vi "ni579x Wait for EEPROM Operation.vi"(0 "Register Bus":T1, 1 "scope":string(combo)="characterization data eeprom", 9 "timeout [s]":dbl=10.0, 11 "Error In":errorcluster) -> (4 "Register Bus (out)":T1, 15 "Error Out":errorcluster)   [LabVIEW 2015, in "ni579x Config v2 Host.lvlib"]
uses:
  <instrlib>/ni579x/Config/v2/Host/ni579x Config v2 Host.lvlib
  <instrlib>/_niInstr/Register Bus/v0/Host/Public/Register Bus Session.ctl
  <instrlib>/_niInstr/Register Bus/v0/Host/Private/Session Data.ctl
  <instrlib>/ni579x/Config/v2/Shared/Types/ni579x FAM Register Offset.ctl
  <instrlib>/ni579x/Config/v2/Shared/Types/ni579x FAM Register Operation.ctl
  <instrlib>/ni579x/Config/v2/Shared/ni579x Config v2 Shared.lvlib
  <instrlib>/_niInstr/Register Bus/v0/Host/niInstr Register Bus v0 Host.lvlib
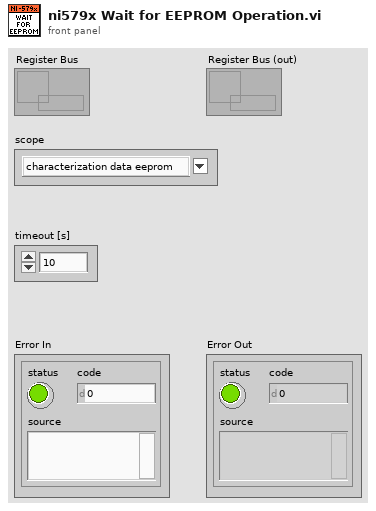
[diagram p1: front panel]
types:
  T1 = typedef "niInstr Register Bus v0 Host.lvlib/Register Bus Session.ctl" = refnum<queue>
  T2 = typedef "ni579x Config v2 Shared.lvlib/ni579x FAM Register Operation.ctl" = cluster{"FAM Register Offset":T3, "Address":u32, "Write (T)/Read (F)":bool, "Write Data":u32}
  T3 = typedef "ni579x Config v2 Shared.lvlib/ni579x FAM Register Offset.ctl" = u8
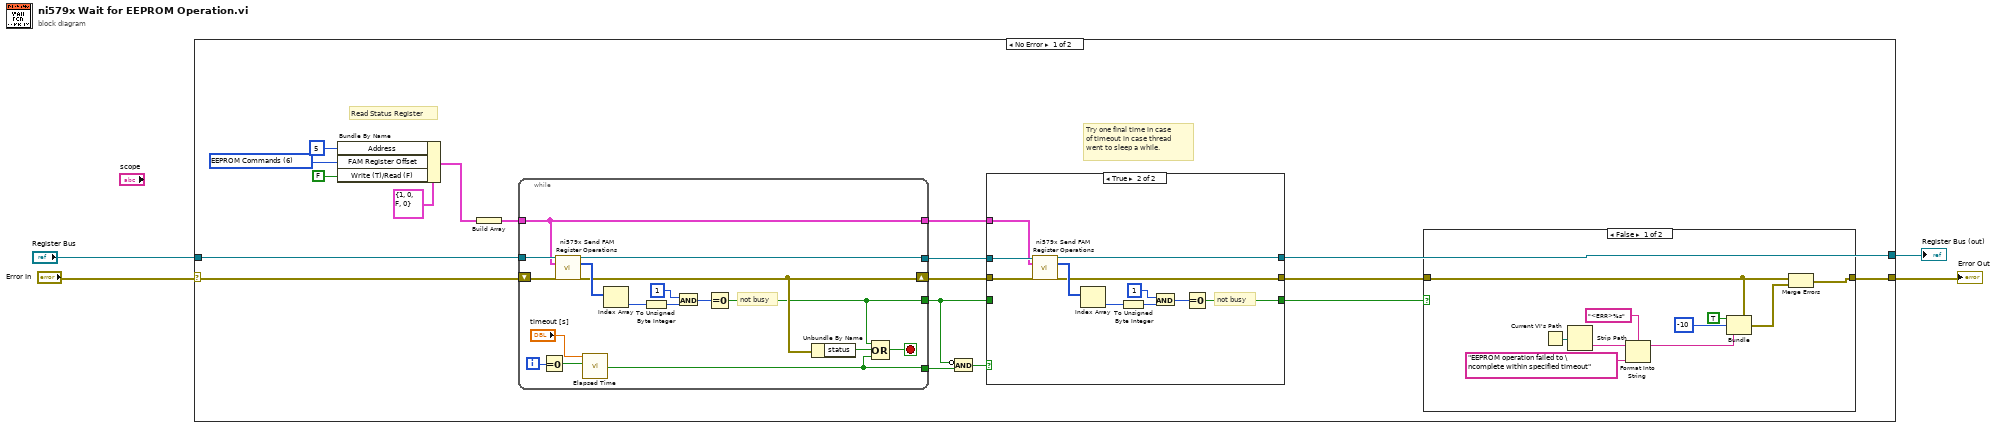
[diagram p0: block diagram]
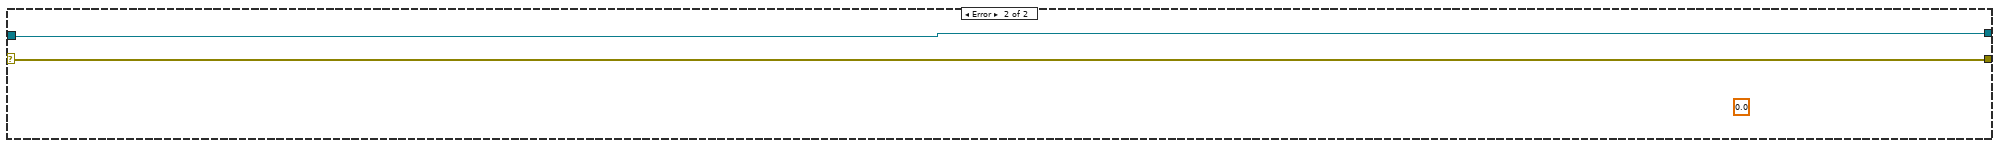
[diagram p4: hidden frame]
diagram:
  n1 = case shown="No Error" "Error In" {
    selector: "Error In" -> [w10 w66]
    tunnel: [w17 w66] -> w3
    tunnel: "Register Bus" -> [w12 w65]
    tunnel: [w7 w65] -> w1
    frame No Error {
      w6 = T3 6 items=["ADC"=1, "DAC"=2, "Clock Distribution Chip"=3, "Frequency/Phase Adjust DAC"=4, "EEPROM"=5, "EEPROM Commands"=6, "LO1"=7, "Rx Atten Pre-LNA"=9, "Rx Atten Post-LNA"=10, "Tx Atten"=11] ("FAM Register Offset")
      # "Try one final time in case\nof timeout in case thread\nwent to sleep a while."
      # "Read Status Register"
      n2 = Bundle By Name(cluster=T2 {"FAM Register Offset"=1, "Address"=0, "Write (T)/Read (F)"=FALSE, "Write Data"=0} ("FAM Register Operation"), "Address"=u32 5, "FAM Register Offset"=w6, "Write (T)/Read (F)"=FALSE) -> (w15:T2)
      n3 = Build Array(w15) -> (w11:T2[])
      n4 = while {
        shift-right: [w52] -> w20
        shift-left: w10 -> [w57]
        tunnel: [w61] -> w22
        tunnel: [w50] -> w16
        tunnel: w12 -> [w58]
        tunnel: w11 -> [w48]
        tunnel: [w49] -> w9
        tunnel: [w48] -> w8
        i -> [w63]
        stop <- w62 stop-if-true
        # "not busy"
        n5 = Equal To 0?(x=w63) -> (x = 0?=w64:bool)
        n6 = call <instrlib>:"ni579x Send FAM Register Operations.vi"("Register Bus"=w58, "FAM Register Operations"=w48, "Error In"=w57) -> ("Register Bus (out)"=w49:T1, "FAM Register Read Data"=w56:u32[], "Error Out"=w52:errorcluster)  [unwired: 10 in]
        n7 = call "Elapsed Time"("Time Target (s)"="timeout [s]", "Reset"=w64) -> ("Time has Elapsed"=w61:bool)  [unwired: 10 in, 7 out]
        n8 = Index Array(array=w56) -> (element=w55:u32)  [unwired: 1 in]
        n9 = To Unsigned Byte Integer(number=w55) -> (unsigned 8bit integer=w54:u8)
        n10 = And(x=u8 1, y=w54) -> (x .and. y?=w51:u8)
        n11 = Equal To 0?(x=w51) -> (x = 0?=w50:bool)
        n12 = Unbundle By Name(w52) -> ("status"=w59:bool)
        n13 = Compound Arithmetic op=OR(w50, w59, w61) -> (w62:bool)
      }
      n14 = Compound Arithmetic op=AND(invert w16, w22) -> (w21:bool)
      n15 = case shown="True" w21 {
        tunnel: w20 -> [w25 w31]
        tunnel: [w24 w27] -> w19
        tunnel: [w25 w28] -> w18
        tunnel: w16 -> [w24 _]
        tunnel: w9 -> [w23 w30]
        tunnel: w8 -> [_ w29]
        tunnel: [w23 w26] -> w7
        frame False {
        }
        frame True {
          # "not busy"
          n16 = call <instrlib>:"ni579x Send FAM Register Operations.vi"("Register Bus"=w30, "FAM Register Operations"=w29, "Error In"=w31) -> ("Register Bus (out)"=w26:T1, "FAM Register Read Data"=w36:u32[], "Error Out"=w28:errorcluster)  [unwired: 10 in]
          n17 = Index Array(array=w36) -> (element=w35:u32)  [unwired: 1 in]
          n18 = To Unsigned Byte Integer(number=w35) -> (unsigned 8bit integer=w34:u8)
          n19 = And(x=u8 1, y=w34) -> (x .and. y?=w32:u8)
          n20 = Equal To 0?(x=w32) -> (x = 0?=w27:bool)
        }
      }
      n21 = case shown="False" w19 {
        tunnel: w18 -> [w38 w47]
        tunnel: [w37 w47] -> w17
        frame False {
          n22 = Current VI's Path() -> (path=w45:path)
          n23 = Strip Path(path=w45) -> (name=w44:string)  [unwired: 1 out]
          n24 = Format Into String(format string="<ERR>%s", initial string=w44, "EEPROM operation failed to \ncomplete within specified timeout" ("input 1")) -> (resulting string=w43:string)  [unwired: 1 in, 1 out]
          n25 = Bundle(cluster=w38, "status"=TRUE, "code"=-10, "source"=w43) -> (w42:errorcluster)
          n26 = Merge Errors(w38, w42) -> (w37:errorcluster)
        }
        frame True {
        }
      }
    }
    frame Error {
      (unwired) 0.0 ("coerced attenuation [dB]")
    }
  }
  "Register Bus (out)" <- w1
  "Error Out" <- w3
